vi "updateSetPoint.vi"(8 "error in (no error)":errorcluster, 10 "new setpoint":dbl, 11 "PIDController in":refnum<class "PIDController.lvclass">) -> (0 "error out":errorcluster, 3 "PIDController out":refnum<class "PIDController.lvclass">)   [LabVIEW 2025, in "PIDController.lvclass"]
uses:
  PIDController.lvclass
  PIDController.lvclass/PIDController.ctl
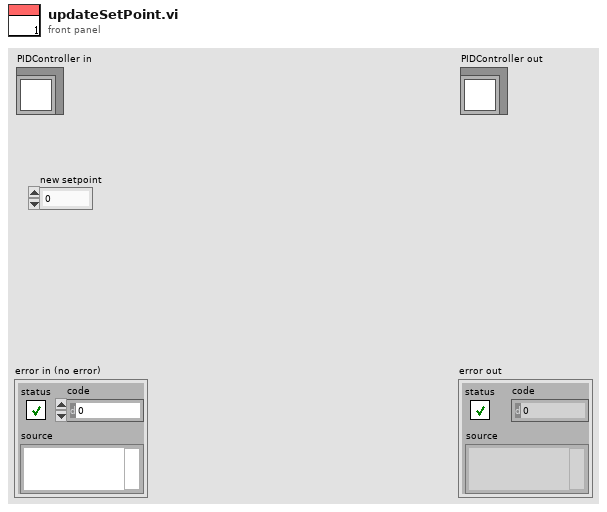
[diagram p1: front panel]
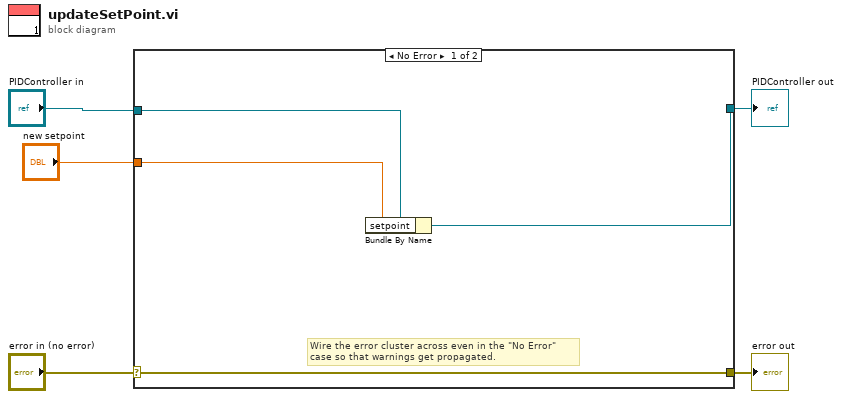
[diagram p0: block diagram]
diagram:
  n1 = case shown="No Error" "error in (no error)" {
    selector: "error in (no error)" -> [w9 w11]
    tunnel: [w9 w11] -> w4
    tunnel: [w8 w10] -> w2
    tunnel: "PIDController in" -> [w6 w10]
    tunnel: "new setpoint" -> [w7 _]
    frame No Error {
      # "Wire the error cluster across even in the \"No Error\"\ncase so that warnings get propagated."
      n2 = Bundle By Name(cluster=w6, "setpoint"=w7) -> (w8:refnum<class "PIDController.lvclass">)
    }
    frame Error {
    }
  }
  "error out" <- w4
  "PIDController out" <- w2
